vi "DriverStationGetData.vi"   [LabVIEW 2020]
doc: "This VI recieves data from the FRC 4265 Dashboard continuously, in all robot modes. These may include safety overrides, calibration commands, and configuration parameters. However this VI should never include standard driver or manipulator commands."
uses:
  f2972b46-d919-4210-bfdf-d3cf9c7f3ddc.vi
  GlobalDriverStationData.vi
  <vilib>/Rock Robotics/Network Tables/NT Read Number.vi
  <vilib>/Rock Robotics/Network Tables/NT Read Boolean.vi
  GlobalDrivebase.vi
  GlobalArm.vi
  GlobalPoseAndTargeting.vi
  <vilib>/Rock Robotics/Network Tables/NT Read String.vi
  <vilib>/Rock Robotics/Network Tables/NT Read Numeric Array.vi
  GlobalDriverStationCommands.vi
  GRNF_Joystick.vi
  <vilib>/Utility/xml.llb/Write to XML File(string).vi
types:
  T1 = enum16{"Center", "North", "NorthWest", "West", "SouthWest", "South", "SouthEast", "East", "NorthEast"}
  T2 = typedef "WPI_JoystickDevRef.ctl" = cluster{"Device":T3}
  T3 = typedef "WPI_JoystickDeviceEnum.ctl" = enum16{"USB 0", "USB 1", "USB 2", "USB 3", "USB 4", "USB 5"}
  T4 = typedef "WPI_DriverStationAllianceInfo.ctl" = enum16{"Red", "Blue", "Invalid"}
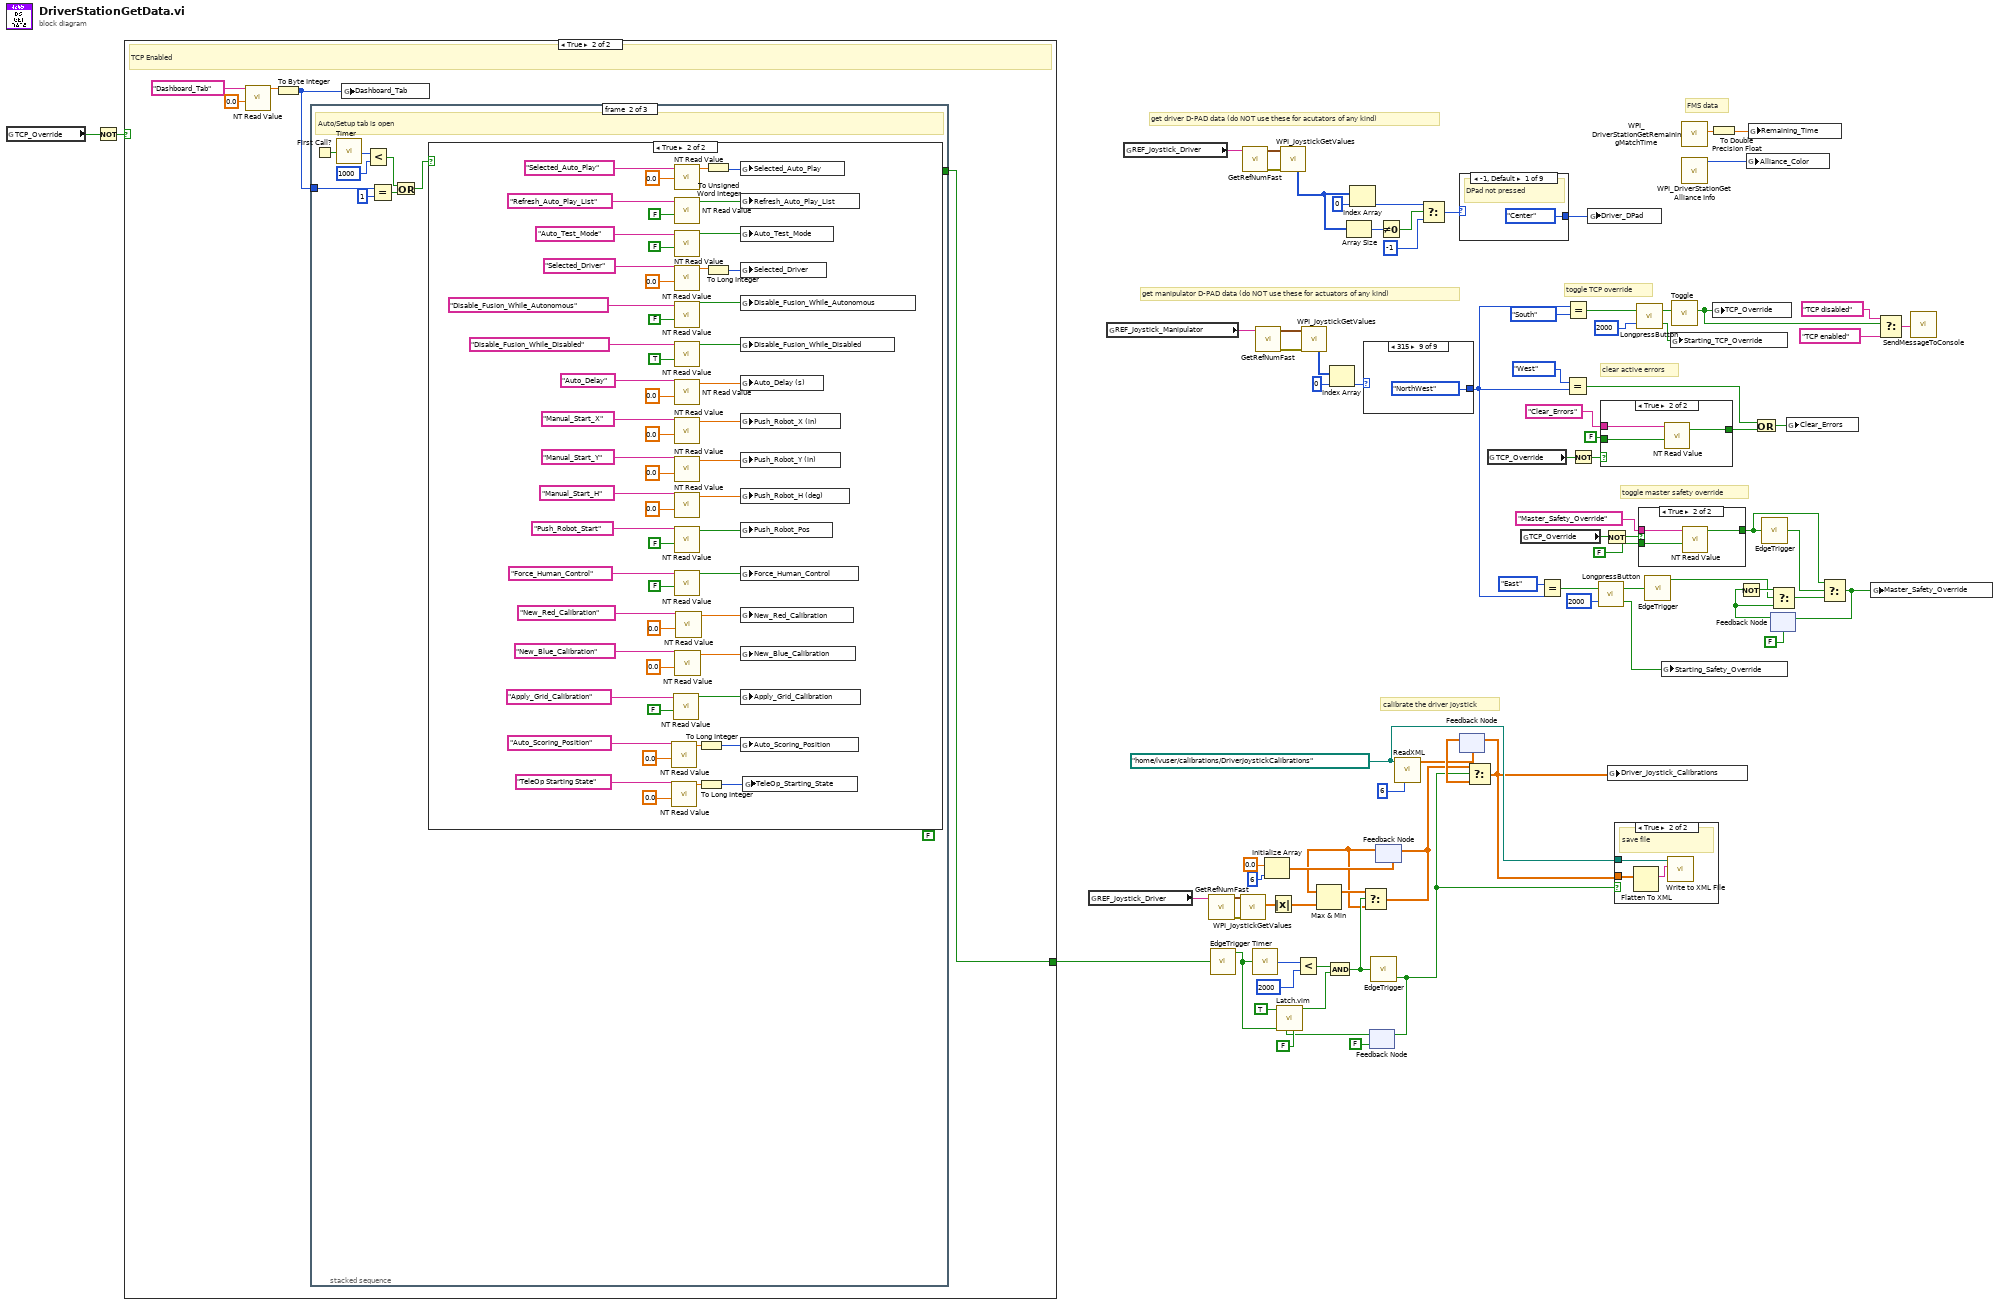
[diagram p0: block diagram]
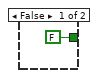
[diagram p2: hidden frame]
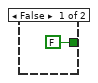
[diagram p3: hidden frame]
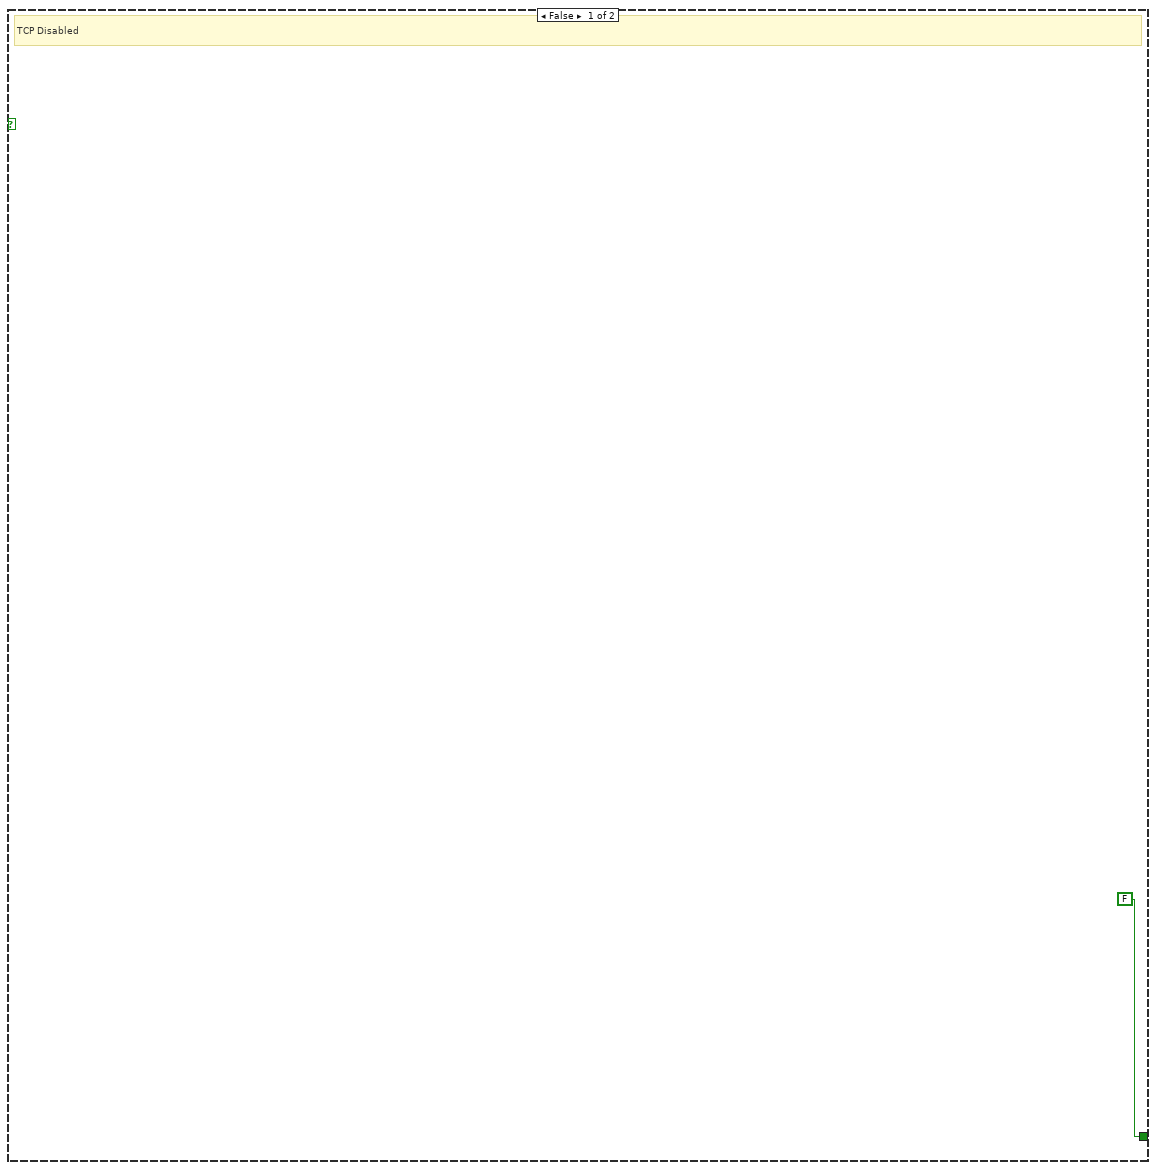
[diagram p4: hidden frame]
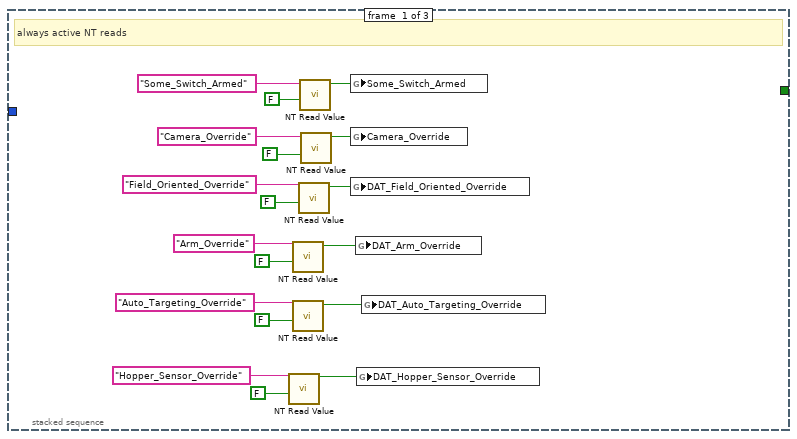
[diagram p5: hidden frame]
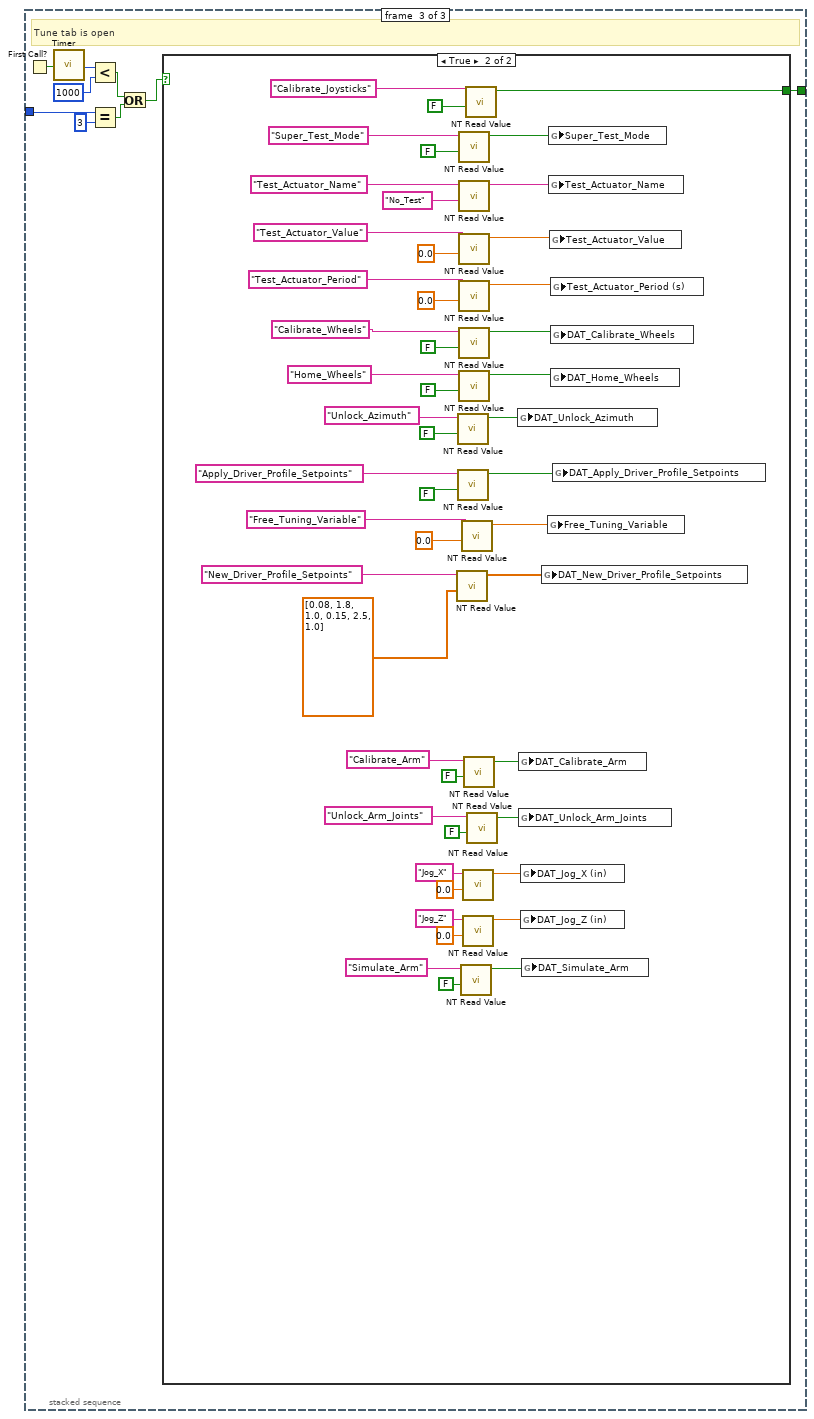
[diagram p7: hidden frame]
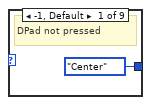
[diagram p9: hidden frame]
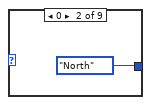
[diagram p10: hidden frame]
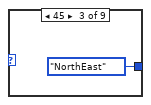
[diagram p11: hidden frame]
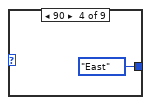
[diagram p12: hidden frame]
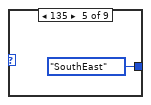
[diagram p13: hidden frame]
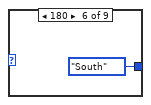
[diagram p14: hidden frame]
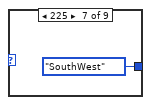
[diagram p15: hidden frame]
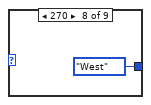
[diagram p16: hidden frame]
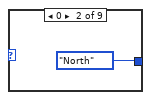
[diagram p17: hidden frame]
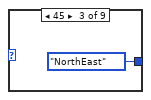
[diagram p18: hidden frame]
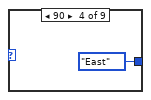
[diagram p19: hidden frame]
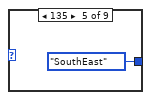
[diagram p20: hidden frame]
diagram:
  w82 = path "/home/lvuser/calibrations/DriverJoystickCalibrations" ("path")
  # "toggle master safety override"
  # "clear active errors"
  # "toggle TCP override"
  # "FMS data"
  # "get manipulator D-PAD data (do NOT use these for actuators of any kind)"
  # "get driver D-PAD data (do NOT use these for acutators of any kind)"
  # "calibrate the driver joystick"
  n1 = global read "GlobalDriverStationData.vi" "TCP_Override"() -> (w15:bool)
  n2 = Not(x=w15) -> (.not. x?=w14:bool)
  n3 = case shown="True" w14 {
    tunnel: [FALSE ("Boolean") w87] -> w26
    frame False {
      # "TCP Disabled"
    }
    frame True {
      # "TCP Enabled"
      n4 = call-poly <vilib>:"NT Read Value.vi"("default value"=0.0 ("Default Value"), "name"="Dashboard_Tab" ("refnum name")) -> ("value"=w89:dbl)  [unwired: 7 in, 2 out]
      n5 = To Byte Integer(number=w89) -> (8bit integer=w88:i8)
      n6 = stacked-sequence {
        tunnel: w88 -> [_ w117 w179]
        tunnel: [_ _ w177] -> w87
        frame #0 {
          # "always active NT reads"
          n7 = call-poly <vilib>:"NT Read Value.vi"("default value"=FALSE ("Default Value"), "name"="Hopper_Sensor_Override" ("refnum name")) -> ("value"=w92:bool)  [unwired: 7 in, 2 out]
          n8 = call-poly <vilib>:"NT Read Value.vi"("default value"=FALSE ("Default Value"), "name"="Arm_Override" ("refnum name")) -> ("value"=w98:bool)  [unwired: 7 in, 2 out]
          n9 = call-poly <vilib>:"NT Read Value.vi"("default value"=FALSE ("Default Value"), "name"="Auto_Targeting_Override" ("refnum name")) -> ("value"=w95:bool)  [unwired: 7 in, 2 out]
          n10 = call-poly <vilib>:"NT Read Value.vi"("default value"=FALSE ("Default Value"), "name"="Field_Oriented_Override" ("refnum name")) -> ("value"=w101:bool)  [unwired: 7 in, 2 out]
          n11 = call-poly <vilib>:"NT Read Value.vi"("default value"=FALSE ("Default Value"), "name"="Some_Switch_Armed" ("refnum name")) -> ("value"=w109:bool)  [unwired: 7 in, 2 out]
          n12 = call-poly <vilib>:"NT Read Value.vi"("default value"=FALSE ("Default Value"), "name"="Camera_Override" ("refnum name")) -> ("value"=w106:bool)  [unwired: 7 in, 2 out]
          n13 = global write "GlobalDriverStationData.vi" "Some_Switch_Armed"(w109) -> ()
          n14 = global write "GlobalDriverStationData.vi" "Camera_Override"(w106) -> ()
          n15 = global write "GlobalDrivebase.vi" "DAT_Field_Oriented_Override"(w101) -> ()
          n16 = global write "GlobalArm.vi" "DAT_Arm_Override"(w98) -> ()
          n17 = global write "GlobalDrivebase.vi" "DAT_Hopper_Sensor_Override"(w92) -> ()
          n18 = global write "GlobalDrivebase.vi" "DAT_Auto_Targeting_Override"(w95) -> ()
        }
        frame #1 {
          (unwired) FALSE ("Boolean")
          # "Auto/Setup tab is open"
          n19 = First Call?() -> (First Call?: T/F=w115:bool)
          n20 = call "Timer.vi"("Reset Timer"=w115) -> ("Time (ms)"=w114:u32)
          n21 = Less?(x=w114, y=u32 1000 ("Time threshold (ms)")) -> (x < y?=w112:bool)
          n22 = Equal?(x=w117, y=i8 1) -> (x = y?=w113:bool)
          n23 = Or(x=w112, y=w113) -> (x .or. y?=w111:bool)
          n24 = case shown="True" w111 {
            frame False {
            }
            frame True {
              n25 = call-poly <vilib>:"NT Read Value.vi"("default value"=0.0 ("Default Value"), "name"="Auto_Scoring_Position" ("refnum name")) -> ("value"=w123:dbl)  [unwired: 7 in, 2 out]
              n26 = call-poly <vilib>:"NT Read Value.vi"("default value"=0.0 ("Default Value"), "name"="TeleOp Starting State" ("refnum name")) -> ("value"=w119:dbl)  [unwired: 7 in, 2 out]
              n27 = call-poly <vilib>:"NT Read Value.vi"("default value"=FALSE ("Default Value"), "name"="Apply_Grid_Calibration" ("refnum name")) -> ("value"=w126:bool)  [unwired: 7 in, 2 out]
              n28 = call-poly <vilib>:"NT Read Value.vi"("default value"=0.0 ("Default Value"), "name"="Selected_Auto_Play" ("refnum name")) -> ("value"=w161:dbl)  [unwired: 7 in, 2 out]
              n29 = call-poly <vilib>:"NT Read Value.vi"("default value"=FALSE ("Default Value"), "name"="Refresh_Auto_Play_List" ("refnum name")) -> ("value"=w160:bool)  [unwired: 7 in, 2 out]
              n30 = call-poly <vilib>:"NT Read Value.vi"("default value"=FALSE ("Default Value"), "name"="Auto_Test_Mode" ("refnum name")) -> ("value"=w172:bool)  [unwired: 7 in, 2 out]
              n31 = call-poly <vilib>:"NT Read Value.vi"("default value"=0.0 ("Default Value"), "name"="Selected_Driver" ("refnum name")) -> ("value"=w163:dbl)  [unwired: 7 in, 2 out]
              n32 = call-poly <vilib>:"NT Read Value.vi"("default value"=FALSE ("Default Value"), "name"="Disable_Fusion_While_Autonomous" ("refnum name")) -> ("value"=w166:bool)  [unwired: 7 in, 2 out]
              n33 = call-poly <vilib>:"NT Read Value.vi"("default value"=TRUE ("Default Value"), "name"="Disable_Fusion_While_Disabled" ("refnum name")) -> ("value"=w167:bool)  [unwired: 7 in, 2 out]
              n34 = call-poly <vilib>:"NT Read Value.vi"("default value"=0.0 ("Default Value"), "name"="Auto_Delay" ("refnum name")) -> ("value"=w165:dbl)  [unwired: 7 in, 2 out]
              n35 = call-poly <vilib>:"NT Read Value.vi"("default value"=0.0 ("Default Value"), "name"="Manual_Start_X" ("refnum name")) -> ("value"=w168:dbl)  [unwired: 7 in, 2 out]
              n36 = call-poly <vilib>:"NT Read Value.vi"("default value"=0.0 ("Default Value"), "name"="Manual_Start_Y" ("refnum name")) -> ("value"=w169:dbl)  [unwired: 7 in, 2 out]
              n37 = call-poly <vilib>:"NT Read Value.vi"("default value"=0.0 ("Default Value"), "name"="Manual_Start_H" ("refnum name")) -> ("value"=w170:dbl)  [unwired: 7 in, 2 out]
              n38 = call-poly <vilib>:"NT Read Value.vi"("default value"=FALSE ("Default Value"), "name"="Push_Robot_Start" ("refnum name")) -> ("value"=w171:bool)  [unwired: 7 in, 2 out]
              n39 = call-poly <vilib>:"NT Read Value.vi"("default value"=FALSE ("Default Value"), "name"="Force_Human_Control" ("refnum name")) -> ("value"=w137:bool)  [unwired: 7 in, 2 out]
              n40 = call-poly <vilib>:"NT Read Value.vi"("default value"=0.0 ("Default Value"), "name"="New_Blue_Calibration" ("refnum name")) -> ("value"=w129:dbl)  [unwired: 7 in, 2 out]
              n41 = call-poly <vilib>:"NT Read Value.vi"("default value"=0.0 ("Default Value"), "name"="New_Red_Calibration" ("refnum name")) -> ("value"=w132:dbl)  [unwired: 7 in, 2 out]
              n42 = To Long Integer(number=w123) -> (32bit integer=w122:i32)
              n43 = To Long Integer(number=w119) -> (32bit integer=w118:i32)
              n44 = To Unsigned Word Integer(number=w161) -> (unsigned 16bit integer=w162:u16)
              n45 = To Long Integer(number=w163) -> (32bit integer=w164:i32)
              n46 = global write "GlobalDriverStationData.vi" "Selected_Auto_Play"(w162) -> ()
              n47 = global write "GlobalDriverStationData.vi" "Refresh_Auto_Play_List"(w160) -> ()
              n48 = global write "GlobalDriverStationData.vi" "Auto_Test_Mode"(w172) -> ()
              n49 = global write "GlobalDriverStationData.vi" "Selected_Driver"(w164) -> ()
              n50 = global write "GlobalDriverStationData.vi" "Disable_Fusion_While_Autonomous"(w166) -> ()
              n51 = global write "GlobalDriverStationData.vi" "Disable_Fusion_While_Disabled"(w167) -> ()
              n52 = global write "GlobalDriverStationData.vi" "Auto_Delay (s)"(w165) -> ()
              n53 = global write "GlobalPoseAndTargeting.vi" "Push_Robot_X (in)"(w168) -> ()
              n54 = global write "GlobalPoseAndTargeting.vi" "Push_Robot_Y (in)"(w169) -> ()
              n55 = global write "GlobalPoseAndTargeting.vi" "Push_Robot_H (deg)"(w170) -> ()
              n56 = global write "GlobalPoseAndTargeting.vi" "Push_Robot_Pos"(w171) -> ()
              n57 = global write "GlobalDriverStationData.vi" "Force_Human_Control"(w137) -> ()
              n58 = global write "GlobalPoseAndTargeting.vi" "New_Red_Calibration"(w132) -> ()
              n59 = global write "GlobalPoseAndTargeting.vi" "New_Blue_Calibration"(w129) -> ()
              n60 = global write "GlobalPoseAndTargeting.vi" "Apply_Grid_Calibration"(w126) -> ()
              n61 = global write "GlobalDriverStationData.vi" "Auto_Scoring_Position"(w122) -> ()
              n62 = global write "GlobalDriverStationData.vi" "TeleOp_Starting_State"(w118) -> ()
            }
          }
        }
        frame #2 {
          # "Tune tab is open"
          n63 = First Call?() -> (First Call?: T/F=w176:bool)
          n64 = call "Timer.vi"("Reset Timer"=w176) -> ("Time (ms)"=w175:u32)
          n65 = Less?(x=w175, y=u32 1000 ("Time threshold (ms)")) -> (x < y?=w173:bool)
          n66 = Equal?(x=w179, y=i8 3) -> (x = y?=w181:bool)
          n67 = Or(x=w173, y=w181) -> (x .or. y?=w178:bool)
          n68 = case shown="True" w178 {
            tunnel: [_ w204] -> w177
            frame False {
            }
            frame True {
              n69 = call-poly <vilib>:"NT Read Value.vi"("default value"=dbl[] [0.08, 1.8, 1.0, 0.15, 2.5, 1.0] ("Default Value"), "name"="New_Driver_Profile_Setpoints" ("Name")) -> ("value"=w200:dbl[])  [unwired: 7 in, 2 out]
              n70 = call-poly <vilib>:"NT Read Value.vi"("default value"=FALSE ("Default Value"), "name"="Unlock_Azimuth" ("refnum name")) -> ("value"=w182:bool)  [unwired: 7 in, 2 out]
              n71 = call-poly <vilib>:"NT Read Value.vi"("default value"=FALSE ("Default Value"), "name"="Apply_Driver_Profile_Setpoints" ("Name")) -> ("value"=w201:bool)  [unwired: 7 in, 2 out]
              n72 = call-poly <vilib>:"NT Read Value.vi"("default value"=FALSE ("Default Value"), "name"="Super_Test_Mode" ("refnum name")) -> ("value"=w229:bool)  [unwired: 7 in, 2 out]
              n73 = call-poly <vilib>:"NT Read Value.vi"("default value"="No_Test" ("Default Value"), "name"="Test_Actuator_Name" ("refnum name")) -> ("value"=w224:string)  [unwired: 7 in, 2 out]
              n74 = call-poly <vilib>:"NT Read Value.vi"("default value"=0.0 ("Default Value"), "name"="Test_Actuator_Value" ("refnum name")) -> ("value"=w225:dbl)  [unwired: 7 in, 2 out]
              n75 = call-poly <vilib>:"NT Read Value.vi"("default value"=0.0 ("Default Value"), "name"="Test_Actuator_Period" ("refnum name")) -> ("value"=w226:dbl)  [unwired: 7 in, 2 out]
              n76 = call-poly <vilib>:"NT Read Value.vi"("default value"=FALSE ("Default Value"), "name"="Calibrate_Wheels" ("refnum name")) -> ("value"=w203:bool)  [unwired: 7 in, 2 out]
              n77 = call-poly <vilib>:"NT Read Value.vi"("default value"=FALSE ("Default Value"), "name"="Home_Wheels" ("refnum name")) -> ("value"=w202:bool)  [unwired: 7 in, 2 out]
              n78 = call-poly <vilib>:"NT Read Value.vi"("default value"=FALSE ("Default Value"), "name"="Simulate_Arm" ("Name")) -> ("value"=w185:bool)  [unwired: 7 in, 2 out]
              n79 = call-poly <vilib>:"NT Read Value.vi"("default value"=0.0 ("Default Value"), "name"="Free_Tuning_Variable" ("refnum name")) -> ("value"=w210:dbl)  [unwired: 7 in, 2 out]
              n80 = call-poly <vilib>:"NT Read Value.vi"("default value"=0.0, "name"="Jog_X" ("Name")) -> ("value"=w192:dbl)  [unwired: 7 in, 2 out]
              n81 = call-poly <vilib>:"NT Read Value.vi"("default value"=0.0, "name"="Jog_Z" ("Name")) -> ("value"=w190:dbl)  [unwired: 7 in, 2 out]
              n82 = call-poly <vilib>:"NT Read Value.vi"("default value"=FALSE ("Default Value"), "name"="Calibrate_Arm" ("Name")) -> ("value"=w197:bool)  [unwired: 7 in, 2 out]
              n83 = call-poly <vilib>:"NT Read Value.vi"("default value"=FALSE ("Default Value"), "name"="Calibrate_Joysticks" ("refnum name")) -> ("value"=w204:bool)  [unwired: 7 in, 2 out]
              n84 = call-poly <vilib>:"NT Read Value.vi"("default value"=FALSE ("Default Value"), "name"="Unlock_Arm_Joints" ("Name")) -> ("value"=w194:bool)  [unwired: 7 in, 2 out]
              n85 = global write "GlobalDrivebase.vi" "DAT_Unlock_Azimuth"(w182) -> ()
              n86 = global write "GlobalArm.vi" "DAT_Calibrate_Arm"(w197) -> ()
              n87 = global write "GlobalArm.vi" "DAT_Unlock_Arm_Joints"(w194) -> ()
              n88 = global write "GlobalArm.vi" "DAT_Jog_X (in)"(w192) -> ()
              n89 = global write "GlobalArm.vi" "DAT_Jog_Z (in)"(w190) -> ()
              n90 = global write "GlobalArm.vi" "DAT_Simulate_Arm"(w185) -> ()
              n91 = global write "GlobalDrivebase.vi" "DAT_New_Driver_Profile_Setpoints"(w200) -> ()
              n92 = global write "GlobalDriverStationData.vi" "Free_Tuning_Variable"(w210) -> ()
              n93 = global write "GlobalDriverStationData.vi" "Super_Test_Mode"(w229) -> ()
              n94 = global write "GlobalDriverStationData.vi" "Test_Actuator_Name"(w224) -> ()
              n95 = global write "GlobalDriverStationData.vi" "Test_Actuator_Value"(w225) -> ()
              n96 = global write "GlobalDriverStationData.vi" "Test_Actuator_Period (s)"(w226) -> ()
              n97 = global write "GlobalDrivebase.vi" "DAT_Calibrate_Wheels"(w203) -> ()
              n98 = global write "GlobalDrivebase.vi" "DAT_Home_Wheels"(w202) -> ()
              n99 = global write "GlobalDrivebase.vi" "DAT_Apply_Driver_Profile_Setpoints"(w201) -> ()
            }
          }
        }
      }
      n100 = global write "GlobalDriverStationData.vi" "Dashboard_Tab"(w88) -> ()
    }
  }
  n101 = global read "GlobalDriverStationCommands.vi" "REF_Joystick_Driver"() -> (w7:string)
  n102 = global read "GlobalDriverStationCommands.vi" "REF_Joystick_Manipulator"() -> (w8:string)
  n103 = global read "GlobalDriverStationCommands.vi" "REF_Joystick_Driver"() -> (w9:string)
  n104 = call-poly "GetRefNumFast.vi"("RefNum Name"=w7) -> ("Error"=w77:errorcluster, "Device Reference"=w78:T2)  [unwired: 5 in]
  n105 = call "EdgeTrigger.vi"("Input Signal"=w26) -> ("Rising Edge Trigger"=w76:bool)  [unwired: 2 out]
  n106 = call <vilib>:"WPI_JoystickGetValues.vi"("error in (no error)"=w77, "JoystickDevRef"=w78) -> ("Axes"=w66:dbl[])  [unwired: 5 in, 4 out]
  n107 = call-poly "GetRefNumFast.vi"("RefNum Name"=w9) -> ("Error"=w56:errorcluster, "Device Reference"=w57:T2)  [unwired: 5 in]
  n108 = call "Timer.vi"("Reset Timer"=w76) -> ("Time (ms)"=w80:u32)
  n109 = call-poly "GetRefNumFast.vi"("RefNum Name"=w8) -> ("Error"=w84:errorcluster, "Device Reference"=w85:T2)  [unwired: 5 in]
  n110 = Initialize Array(0.0 ("element"), 6 ("dimension size")) -> (w59:dbl[])
  n111 = Absolute Value(x=w66) -> (abs(x)=w63:dbl[])
  n112 = call <vilib>:"WPI_JoystickGetValues.vi"("error in (no error)"=w56, "JoystickDevRef"=w57) -> ("POVs"=w6:i16[])  [unwired: 5 in, 4 out]
  n113 = Less?(x=w80, y=u32 2000) -> (x < y?=w73:bool)
  n114 = call <vilib>:"WPI_JoystickGetValues.vi"("error in (no error)"=w84, "JoystickDevRef"=w85) -> ("POVs"=w51:i16[])  [unwired: 5 in, 4 out]
  n115 = Index Array(array=w51, index=0) -> (element=w52:i16)
  n116 = Array Size(array=w6) -> (size(s)=w5:i32)
  n117 = Index Array(array=w6, index=0) -> (element=w4:i16)
  n118 = case shown="315" w52 {
    tunnel: [T1."Center" T1."North" T1."NorthEast" T1."East" T1."SouthEast" T1."South" T1."SouthWest" T1."West" T1."NorthWest"] -> w24
    frame -1, Default {
      # "DPad not pressed"
    }
    frame 0 {
    }
    frame 45 {
    }
    frame 90 {
    }
    frame 135 {
    }
    frame 180 {
    }
    frame 225 {
    }
    frame 270 {
    }
    frame 315 {
    }
  }
  n119 = feedback #1(FALSE ("Falling Edge Trigger")) -> (w70:bool)
  n120 = call "Latch.vim"("Default Value"=FALSE, "Reset"=w70, "Latch Signal"=w76, "Latch Value"=TRUE) -> ("Latched"=w72:bool)  [unwired: 7 in]
  n121 = And(x=w73, y=w72) -> (x .and. y?=w71:bool)
  n122 = call "EdgeTrigger.vi"("Input Signal"=w71) -> ("Falling Edge Trigger"=w68:bool)  [unwired: 2 out]
  n123 = feedback-in #1(w68) -> ()
  n124 = feedback #2(w59) -> (w58:dbl[])
  n125 = Max & Min(x=w58, y=w63) -> (max(x,y)=w65:dbl[])  [unwired: 1 out]
  n126 = Select(t=w65, s=w71, f=w58) -> (s? t:f=w64:dbl[])
  n127 = feedback-in #2(w64) -> ()
  n128 = Not Equal To 0?(x=w5) -> (x != 0?=w3:bool)
  n129 = call "ReadXML.vi"("Default Number of Elements"=6, "File Path (.xml)"=w82) -> ("Data"=w81:dbl[])  [unwired: 8 in, 1 out]
  n130 = Select(t=w4, s=w3, f=i16 -1) -> (s? t:f=w2:i16)
  n131 = case shown="-1, Default" w2 {
    tunnel: [T1."Center" T1."North" T1."NorthEast" T1."East" T1."SouthEast" T1."South" T1."SouthWest" T1."West" T1."NorthWest"] -> w54
    frame -1, Default {
      # "DPad not pressed"
    }
    frame 0 {
    }
    frame 45 {
    }
    frame 90 {
    }
    frame 135 {
    }
    frame 180 {
    }
    frame 225 {
    }
    frame 270 {
    }
    frame 315 {
    }
  }
  n132 = feedback #3(w81) -> (w83:dbl[])
  n133 = Select(t=w64, s=w68, f=w83) -> (s? t:f=w67:dbl[])
  n134 = feedback-in #3(w67) -> ()
  n135 = global read "GlobalDriverStationData.vi" "TCP_Override"() -> (w11:bool)
  n136 = global read "GlobalDriverStationData.vi" "TCP_Override"() -> (w13:bool)
  n137 = Equal?(x=T1."East", y=w24) -> (x = y?=w40:bool)
  n138 = Equal?(x=T1."West", y=w24) -> (x = y?=w42:bool)
  n139 = Equal?(x=w24, y=T1."South") -> (x = y?=w22:bool)
  n140 = Not(x=w11) -> (.not. x?=w10:bool)
  n141 = global write "GlobalDriverStationData.vi" "Driver_DPad"(w54) -> ()
  n142 = call "LongpressButton.vi"("Threshold (ms)"=u32 2000, "Button"=w40) -> ("Starting Press"=w39:bool, "Longpress Button"=w33:bool)
  n143 = case shown="True" w10 {
    tunnel: FALSE ("Default Value") -> [_ w251]
    tunnel: "Clear_Errors" ("refnum name") -> [_ w250]
    tunnel: [FALSE ("Boolean") w249] -> w43
    frame False {
    }
    frame True {
      n144 = call-poly <vilib>:"NT Read Value.vi"("default value"=w251, "name"=w250) -> ("value"=w249:bool)  [unwired: 7 in, 2 out]
    }
  }
  n145 = Not(x=w13) -> (.not. x?=w12:bool)
  n146 = global write "GlobalDriverStationData.vi" "Driver_Joystick_Calibrations"(w67) -> ()
  n147 = case shown="True" w68 {
    tunnel: w82 -> [_ w254]
    tunnel: w67 -> [_ w253]
    frame False {
    }
    frame True {
      # "save file"
      n148 = Flatten To XML(6:w253) -> (2:w252:string)
      n149 = call-poly <vilib>:"Write to XML File.vi"("XML Input"=w252, "XML File Path"=w254) -> ()  [unwired: 7 in, 3 out]
    }
  }
  n150 = call "LongpressButton.vi"("Threshold (ms)"=u32 2000, "Button"=w22) -> ("Starting Press"=w21:bool, "Longpress Button"=w20:bool)
  n151 = case shown="True" w12 {
    tunnel: FALSE ("Default Value") -> [_ w258]
    tunnel: "Master_Safety_Override" ("refnum name") -> [_ w257]
    tunnel: [FALSE ("Boolean") w256] -> w30
    frame False {
    }
    frame True {
      n152 = call-poly <vilib>:"NT Read Value.vi"("default value"=w258, "name"=w257) -> ("value"=w256:bool)  [unwired: 7 in, 2 out]
    }
  }
  n153 = call "EdgeTrigger.vi"("Input Signal"=w33) -> ("Rising Edge Trigger"=w32:bool)  [unwired: 2 out]
  n154 = global write "GlobalDriverStationData.vi" "Starting_Safety_Override"(w39) -> ()
  n155 = global write "GlobalDriverStationData.vi" "Starting_TCP_Override"(w21) -> ()
  n156 = call "Toggle.vi"("Trigger"=w20) -> ("New State"=w18:bool)  [unwired: 1 in]
  n157 = call <vilib>:"WPI_DriverStationGetRemainingMatchTime.vi"() -> ("Match Time(s)"=w50:sgl)  [unwired: 10 in, 1 out]
  n158 = call <vilib>:"WPI_DriverStationGet Alliance Info.vi"() -> ("Alliance"=w48:T4)  [unwired: 6 in, 5 out]
  n159 = To Double Precision Float(number=w50) -> (double precision float=w49:dbl)
  n160 = global write "GlobalDriverStationData.vi" "TCP_Override"(w18) -> ()
  n161 = global write "GlobalDriverStationData.vi" "Alliance_Color"(w48) -> ()
  n162 = global write "GlobalDriverStationData.vi" "Remaining_Time"(w49) -> ()
  n163 = Or(x=w42, y=w43) -> (x .or. y?=w46:bool)
  n164 = call "EdgeTrigger.vi"("Input Signal"=w30) -> ("All Edge Trigger"=w29:bool)  [unwired: 2 out]
  n165 = feedback #4(FALSE ("Initial State")) -> (w35:bool)
  n166 = Not(x=w35) -> (.not. x?=w36:bool)
  n167 = Select(t=w36, s=w32, f=w35) -> (s? t:f=w31:bool)
  n168 = global write "GlobalDriverStationData.vi" "Clear_Errors"(w46) -> ()
  n169 = Select(t=w30, s=w29, f=w31) -> (s? t:f=w28:bool)
  n170 = feedback-in #4(w28) -> ()
  n171 = global write "GlobalDriverStationData.vi" "Master_Safety_Override"(w28) -> ()
  n172 = Select(t="TCP disabled" ("Message String"), s=w18, f="TCP enabled" ("Message String")) -> (s? t:f=w19:string)
  n173 = call "SendMessageToConsole.vi"("Message String"=w19) -> ()  [unwired: 1 in]
